vi "Luximetro.vi"(0 "Ligado":bool, 3 "Input":dbl) -> (7 "Lux":T1 caption="INTENSIDADE" scale=0.0..10.0 scale format="%#.8p")   [LabVIEW 2018]
uses:
  version_1_interface_luximetro.ctl
panel:
  out "?":bool
  # "Unidade em Lux"
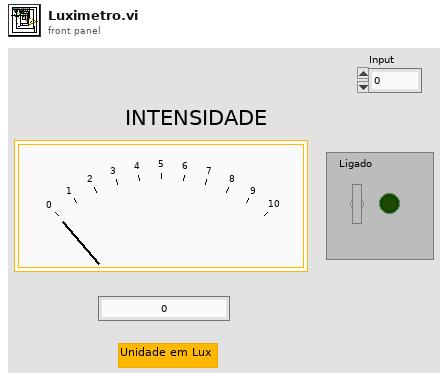
[diagram p1: front panel]
types:
  T1 = typedef "version_1_interface_luximetro.ctl" = dbl
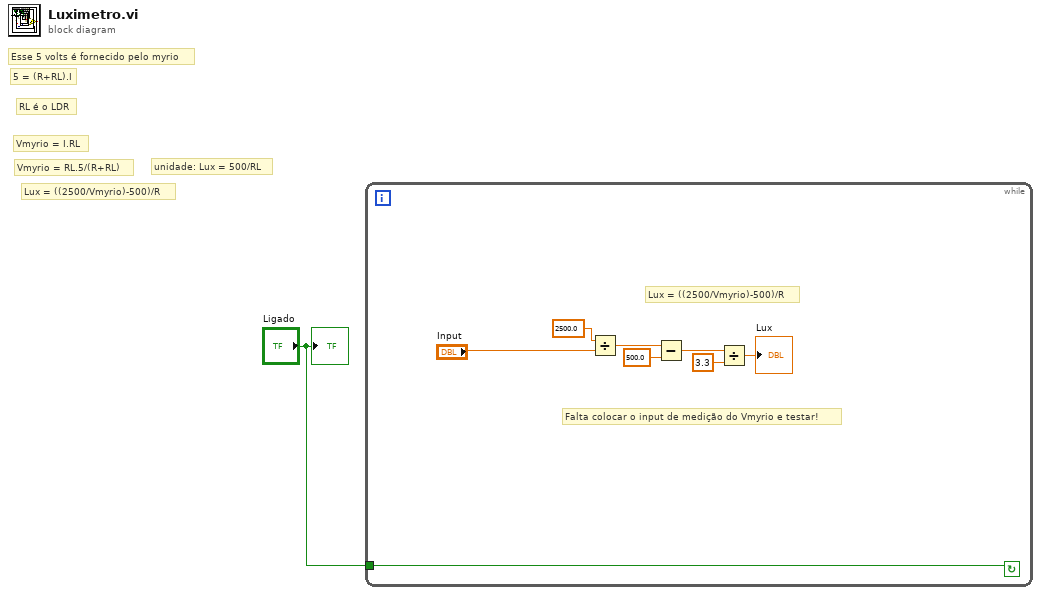
[diagram p0: block diagram]
diagram:
  # "Lux = ((2500/Vmyrio)-500)/R"
  # "RL é o LDR"
  # "Vmyrio = RL.5/(R+RL)"
  # "Esse 5 volts é fornecido pelo myrio"
  # "5 = (R+RL).I"
  # "Vmyrio = I.RL"
  # "unidade: Lux = 500/RL"
  n1 = while {
    tunnel: "Ligado" -> [w9]
    stop <- w9 continue-if-true
    # "Falta colocar o input de medição do Vmyrio e testar!"
    # "Lux = ((2500/Vmyrio)-500)/R"
    n2 = Divide(x=2500.0, y="Input") -> (x/y=w6:dbl)
    n3 = Subtract(x=w6, y=500.0) -> (x-y=w7:dbl)
    n4 = Divide(x=w7, y=3.3) -> (x/y=→"Lux":dbl)
  }
  "?" <- "Ligado"
